vi "SendSMS_TestEACR.vi"(0 "Email Account ID":string, 4 "Port":i32=25, 5 "Email Account Password":string, 7 "SMTP Outgoing Mail Server":string="smtp.gmail.com", 9 "From: (email@site.com)":string, 11 "To: (email@site.com)":string, 12 "Subject:":string, 13 "Body:":string) -> (15 "MailSuccess":bool)   [LabVIEW 2017]
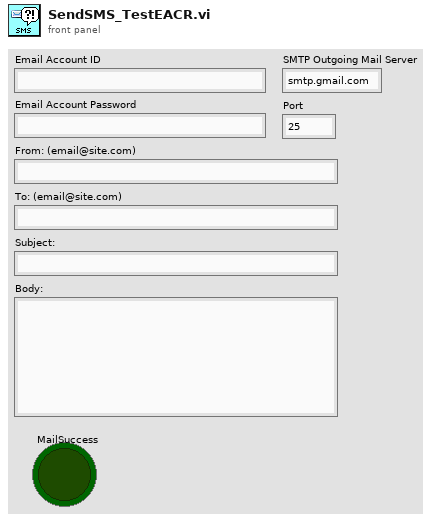
[diagram p1: front panel]
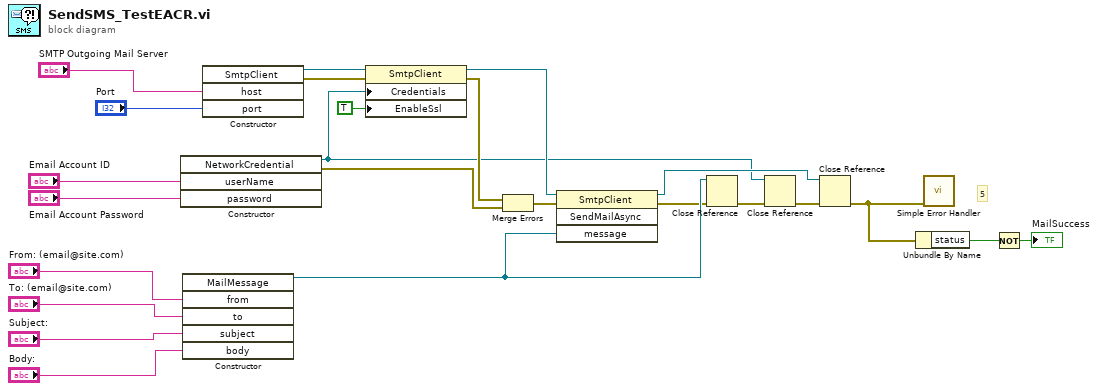
[diagram p0: block diagram]
diagram:
  # "5"
  n1 = constructor class="NetworkCredential"("userName"="Email Account ID", "password"="Email Account Password") -> (reference out=w15:refnum<k24>, error out=w17:errorcluster)  [unwired: 3 in, 3 out]
  n2 = constructor class="MailMessage"("from"="From: (email@site.com)", "to"="To: (email@site.com)", "subject"="Subject:", "body"="Body:") -> (reference out=w12:refnum<k24>)  [unwired: 3 in, 6 out]
  n3 = constructor class="SmtpClient"("host"="SMTP Outgoing Mail Server", "port"="Port") -> (reference out=w24:refnum<k24>, error out=w21:errorcluster)  [unwired: 3 in, 3 out]
  n4 = property class="SmtpClient"(reference=w24, error in=w21, "Credentials"=w15, "EnableSsl"=TRUE ("Enable SSL")) -> (reference out=w23:refnum<k24>, error out=w20:errorcluster)
  n5 = Merge Errors(w20, w17) -> (w19:errorcluster)
  n6 = invoke class="SmtpClient" method="SendMailAsync"(reference=w23, error in=w19, "message"=w12) -> (reference out=w18:refnum<k24>, error out=w10:errorcluster)  [unwired: 1 in, 2 out]
  n7 = Close Reference(reference=w12, error in (no error)=w10) -> (error out=w16:errorcluster)
  n8 = Close Reference(reference=w15, error in (no error)=w16) -> (error out=w14:errorcluster)
  n9 = Close Reference(reference=w18, error in (no error)=w14) -> (error out=w11:errorcluster)
  n10 = Unbundle By Name(w11) -> ("status"=w13:bool)
  n11 = call <vilib>:"Simple Error Handler.vi"("error in (no error)"=w11) -> ()  [unwired: 4 in, 5 out]
  n12 = Not(x=w13) -> (.not. x?=→"MailSuccess":bool)
